vi "Format Client Request (Internal).vi"(8 "error in (no error)":errorcluster, 9 "params":refnum<class "JSON Null.lvclass">, 10 "method":string) -> (0 "error out":errorcluster, 3 "JSON Object out":refnum<class "JSON Object.lvclass">)   [LabVIEW 2015, in "JSONRPC Server.lvclass"]
uses:
  JSONRPC Server.lvclass
  <vilib>/NI/JSON Support for LabVIEW/JSON Data Classes/JSON Datatype/JSON Null.lvclass
  <vilib>/NI/JSON Support for LabVIEW/JSON Data Classes/JSON Object/JSON Object.lvclass
  <vilib>/NI/JSON Support for LabVIEW/JSON Data Classes/JSON Object/New JSON Object (Empty).vi
  <vilib>/NI/JSON Support for LabVIEW/JSON Data Classes/JSON Object/Insert Key Value Pair (Single String).vi
  <vilib>/NI/JSON Support for LabVIEW/JSON Data Classes/JSON Object/Insert Key Value Pair (Single).vi
  <vilib>/NI/JSON Support for LabVIEW/JSON Data Classes/JSON Helper/JSON Helper.lvclass
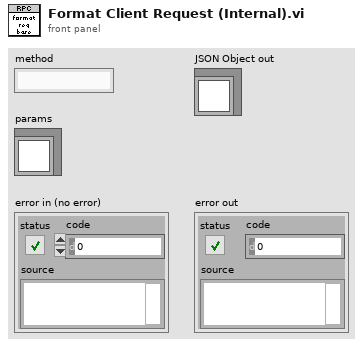
[diagram p1: front panel]
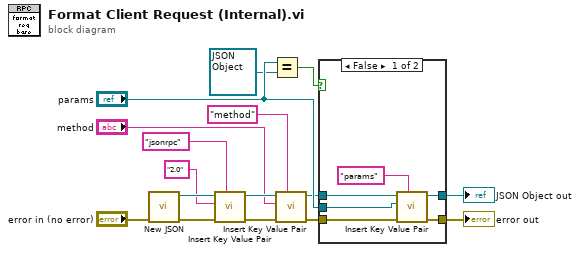
[diagram p0: block diagram]
diagram:
  n1 = call-poly <vilib>:"New JSON.vi"("error in (no error)"="error in (no error)") -> ("error out"=w9:errorcluster, "JSON Object out"=w7:refnum<class "JSON Object.lvclass">)  [unwired: 9 in]
  n2 = call-poly <vilib>:"Insert Key Value Pair.vi"("key"="jsonrpc" ("Name"), "error in (no error)"=w9, "value"="2.0" ("String"), "JSON Object in"=w7) -> ("error out"=w10:errorcluster, "JSON Object out"=w4:refnum<class "JSON Object.lvclass">)  [unwired: 5 in, 1 out]
  n3 = Equal?(x="params", y=refnum<class "JSON Object.lvclass"> refnum ("params")) -> (x = y?=w16:bool)
  n4 = call-poly <vilib>:"Insert Key Value Pair.vi"("key"="method" ("Name"), "error in (no error)"=w10, "value"="method", "JSON Object in"=w4) -> ("error out"=w11:errorcluster, "JSON Object out"=w12:refnum<class "JSON Object.lvclass">)  [unwired: 5 in, 1 out]
  n5 = case shown="False" w16 {
    tunnel: w11 -> [w22 w23]
    tunnel: w12 -> [w19 w24]
    tunnel: [w21 w24] -> w1
    tunnel: [w20 w23] -> w14
    tunnel: "params" -> [w17 _]
    frame False {
      n6 = call-poly <vilib>:"Insert Key Value Pair.vi"("key"="params" ("Name"), "error in (no error)"=w22, "value"=w17, "JSON Object in"=w19) -> ("error out"=w20:errorcluster, "JSON Object out"=w21:refnum<class "JSON Object.lvclass">)  [unwired: 5 in, 1 out]
    }
    frame True {
    }
  }
  "error out" <- w14
  "JSON Object out" <- w1
